vi "Get All Display Areas.vi"(8 "error in (no error)":errorcluster) -> (0 "error out":errorcluster, 3 "Display Areas":T1(array[cluster]))   [LabVIEW 2020, in "MacroAssert.lvlib" / "Win Util.lvlib"]
doc: "Outputs an array of clusters with the horizontal and vertical dimensions in pixels for every display."
uses:
  Win Util.lvlib
  System.Windows.Forms
  System.Drawing
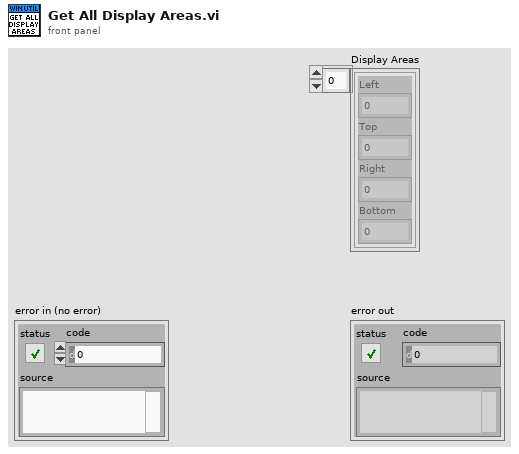
[diagram p1: front panel]
types:
  T1 = cluster{"Left":i32, "Top":i32, "Right":i32, "Bottom":i32}[]
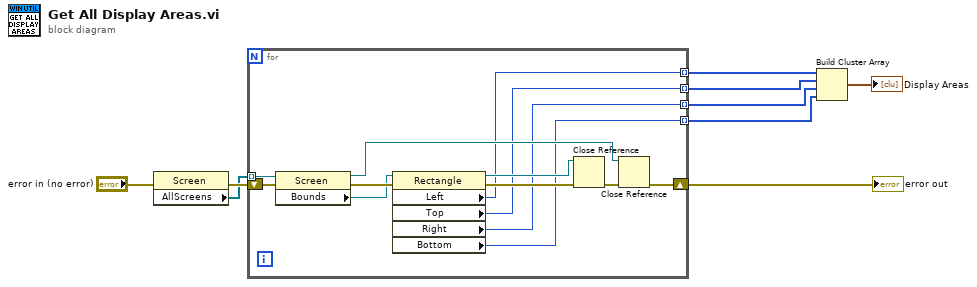
[diagram p0: block diagram]
diagram:
  n1 = property class="Screen"(error in="error in (no error)") -> (error out=w9:errorcluster, "AllScreens"=w7:refnum<k24>[])  [unwired: 1 in, 1 out]
  n2 = for {
    tunnel: w7 -> [w17] mode=indexing
    shift-right: [w15] -> w6
    shift-left: w9 -> [w18]
    tunnel: [w14] -> w2 mode=indexing
    tunnel: [w13] -> w3 mode=indexing
    tunnel: [w12] -> w5 mode=indexing
    tunnel: [w11] -> w4 mode=indexing
    n3 = property class="Screen"(reference=w17, error in=w18) -> (reference out=w21:refnum<k24>, error out=w22:errorcluster, "Bounds"=w10:refnum<k24>)
    n4 = property class="Rectangle"(reference=w10, error in=w22) -> (reference out=w20:refnum<k24>, error out=w19:errorcluster, "Left"=w14:i32, "Top"=w13:i32, "Right"=w12:i32, "Bottom"=w11:i32)
    n5 = Close Reference(reference=w20, error in (no error)=w19) -> (error out=w16:errorcluster)
    n6 = Close Reference(reference=w21, error in (no error)=w16) -> (error out=w15:errorcluster)
  }
  "error out" <- w6
  n7 = Build Cluster Array(w2, w3, w5, w4) -> (→"Display Areas":T1)
